vi "PXI-Enumerate Buffered DIO Lines.vi"(7 "Must be buffered":bool=TRUE, 9 "Must NOT be buffered":bool=TRUE, 11 "error in (no error)":errorcluster) -> (8 "Buffered DIO":tag[](array[tag]), 15 "error out":errorcluster)   [LabVIEW 2020]
uses:
  <resource>/objmgr/daqmx.rc
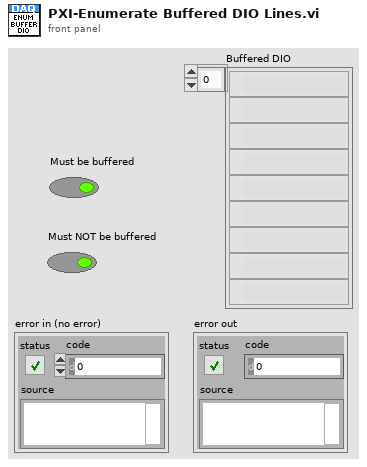
[diagram p1: front panel]
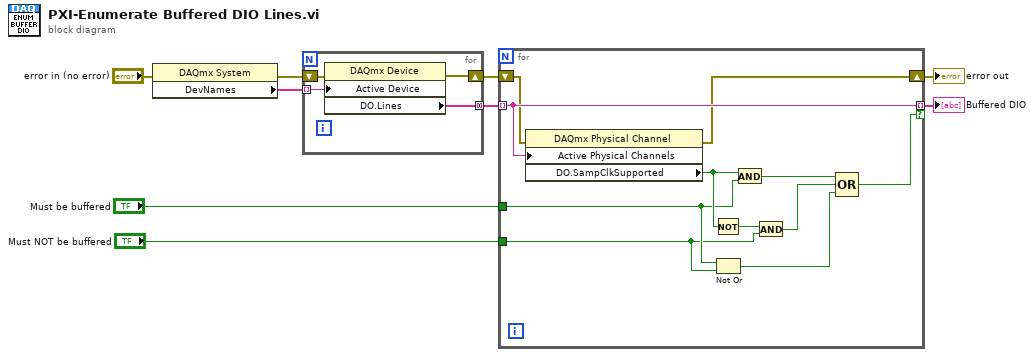
[diagram p0: block diagram]
diagram:
  n1 = property class="DAQmx System"(error in="error in (no error)") -> (error out=w6:errorcluster, "DevNames"=w9:tag[])  [unwired: 1 in, 1 out]
  n2 = for {
    tunnel: w9 -> [w13] mode=indexing
    tunnel: [w12] -> w8 mode=concatenating
    shift-right: [w10] -> w5
    shift-left: w6 -> [w11]
    n3 = property class="DAQmx Device"(error in=w11, "Active Device"=w13) -> (error out=w10:errorcluster, "DO.Lines"=w12:tag[])  [unwired: 1 in, 1 out]
  }
  n4 = for {
    tunnel: w8 -> [w24] mode=indexing
    tunnel: [w24] -> w7 mode=indexing if=w18
    shift-right: [w22] -> w4
    shift-left: w5 -> [w23]
    tunnel: "Must NOT be buffered" -> [w15]
    tunnel: "Must be buffered" -> [w16]
    n5 = property class="DAQmx Physical Channel"(error in=w23, "Active Physical Channels"=w24) -> (error out=w22:errorcluster, "DO.SampClkSupported"=w20:bool)  [unwired: 1 in, 1 out]
    n6 = Not(x=w20) -> (.not. x?=w21:bool)
    n7 = Not Or(1:w15, 2:w16) -> (0:w14:bool)
    n8 = And(x=w20, y=w16) -> (x .and. y?=w19:bool)
    n9 = And(x=w21, y=w15) -> (x .and. y?=w17:bool)
    n10 = Compound Arithmetic op=OR(w19, w17, w14) -> (w18:bool)
  }
  "Buffered DIO" <- w7
  "error out" <- w4
